vi "CalculateRatio.vi"(0 "ratio":dbl, 1 "Cluster":T1={"increase"=0.01, "min velocity"=0.1, "max velocity"=0.4, "Stop increase"=0.01}, 3 "decrease again":bool=TRUE, 5 "velocity":dbl, 7 "acceleration":dbl, 9 "rep":i32, 11 "downramp":dbl, 12 "stop":bool) -> (4 "ratio out":dbl, 6 "velocity out":dbl, 10 "rep out":i32, 14 "decrease again out":bool)   [LabVIEW 2020]
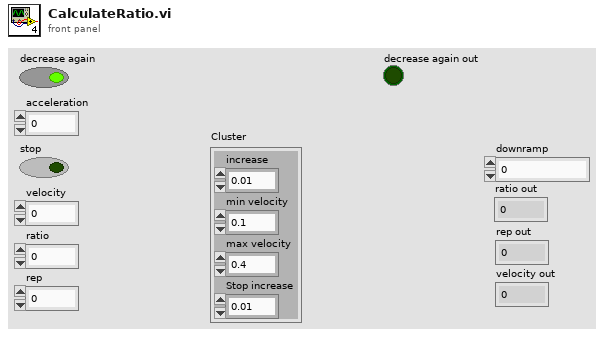
[diagram p1: front panel]
types:
  T1 = cluster{"increase":dbl, "min velocity":dbl, "max velocity":dbl, "Stop increase":dbl}
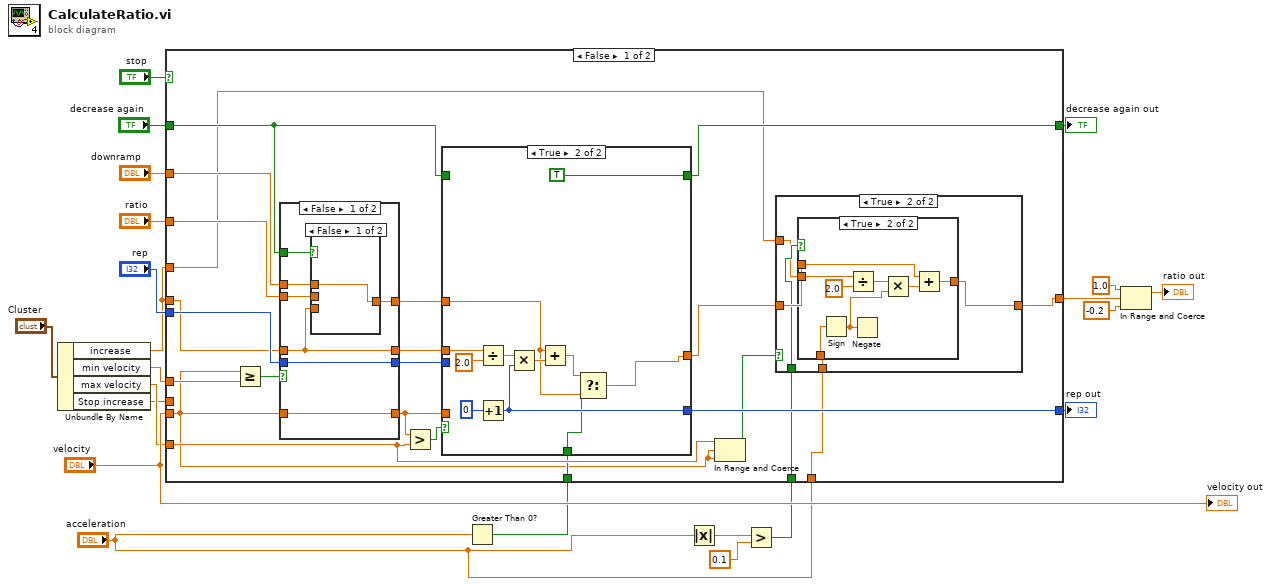
[diagram p0: block diagram]
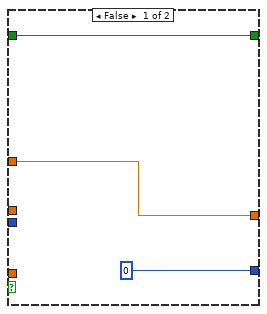
[diagram p4: hidden frame]
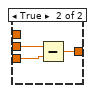
[diagram p5: hidden frame]
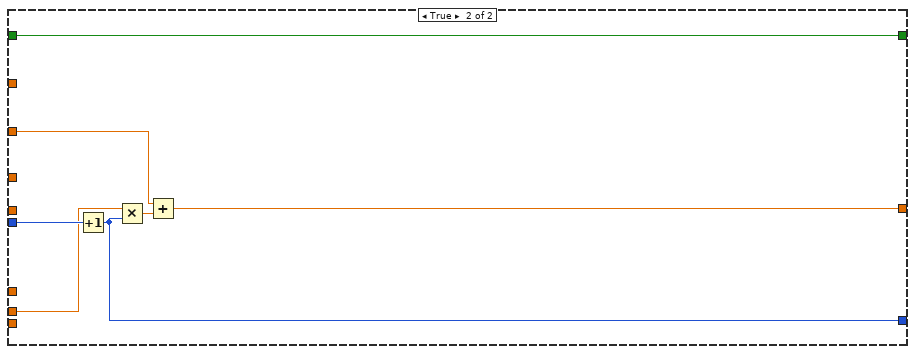
[diagram p7: hidden frame]
diagram:
  n1 = Unbundle By Name("Cluster") -> ("increase"=w1:dbl, "min velocity"=w13:dbl, "max velocity"=w12:dbl, "Stop increase"=w11:dbl)
  n2 = Greater Than 0?(x="acceleration") -> (x > 0?=w6:bool)
  n3 = Absolute Value(x="acceleration") -> (abs(x)=w5:dbl)
  n4 = Greater?(x=w5, y=0.1) -> (0:w3:bool)
  n5 = case shown="False" "stop" {
    tunnel: "velocity" -> [w23 _]
    tunnel: "downramp" -> [w41 _]
    tunnel: "ratio" -> [w40 w96]
    tunnel: [w28 w93] -> w15
    tunnel: "rep" -> [w38 w95]
    tunnel: [w36 w92] -> w9
    tunnel: w1 -> [w35 _]
    tunnel: w13 -> [w34 _]
    tunnel: w12 -> [w31 _]
    tunnel: w11 -> [_ w91]
    tunnel: "decrease again" -> [w32 w90]
    tunnel: [w33 w90] -> w7
    tunnel: w6 -> [w27 _]
    tunnel: w3 -> [w26 _]
    tunnel: "acceleration" -> [w25 _]
    tunnel: w1 -> [w24 _]
    frame False {
      n6 = Greater Or Equal?(x=w23, y=w34) -> (x >= y?=w45:bool)
      n7 = case shown="False" w45 {
        tunnel: w23 -> [w81 w89]
        tunnel: [w81 w89] -> w43
        tunnel: w35 -> [w75 w88]
        tunnel: [w75 w88] -> w42
        tunnel: w41 -> [w79 _]
        tunnel: w40 -> [w76 w87]
        tunnel: [w78 w87] -> w39
        tunnel: w38 -> [w80 w86]
        tunnel: [w80 w86] -> w37
        tunnel: w32 -> [w77 _]
        frame False {
          n8 = case shown="False" w77 {
            tunnel: w79 -> [w82 _]
            tunnel: [w82 w83] -> w78
            tunnel: w76 -> [_ w85]
            tunnel: w75 -> [_ w84]
            frame False {
            }
            frame True {
              n9 = Subtract(x=w85, y=w84) -> (x-y=w83:dbl)
            }
          }
        }
        frame True {
        }
      }
      n10 = Greater?(x=w43, y=w31) -> (0:w44:bool)
      n11 = case shown="True" w44 {
        tunnel: w43 -> [_ _]
        tunnel: w42 -> [_ w74]
        tunnel: [w63 w65] -> w29
        tunnel: w39 -> [w63 w66]
        tunnel: w37 -> [_ _]
        tunnel: [0 w70] -> w36
        tunnel: [w61 TRUE] -> w33
        tunnel: w32 -> [w61 _]
        tunnel: w27 -> [_ w64]
        frame False {
        }
        frame True {
          n12 = Divide(x=w74, y=2.0) -> (x/y=w72:dbl)
          n13 = Increment(x=0) -> (x+1=w70:i32)
          n14 = Multiply(x=w72, y=w70) -> (x*y=w71:dbl)
          n15 = Add(x=w66, y=w71) -> (x+y=w67:dbl)
          n16 = Select(t=w67, s=w64, f=w66) -> (s? t:f=w65:dbl)
        }
      }
      n17 = In Range and Coerce(upper limit=w31, x=w23, lower limit=w23) -> (In Range?=w30:bool)  [unwired: 1 out]
      n18 = case shown="True" w30 {
        tunnel: w29 -> [w46 w51]
        tunnel: [w46 w50] -> w28
        tunnel: w26 -> [_ w49]
        tunnel: w25 -> [_ w48]
        tunnel: w24 -> [_ w47]
        frame False {
        }
        frame True {
          n19 = case shown="True" w49 {
            tunnel: w51 -> [w52 w59]
            tunnel: [w52 w54] -> w50
            tunnel: w48 -> [_ w60]
            tunnel: w47 -> [_ w58]
            frame False {
            }
            frame True {
              n20 = Sign(1:w60) -> (0:w53:dbl)
              n21 = Divide(x=w58, y=2.0) -> (x/y=w56:dbl)
              n22 = Negate(x=w53) -> ()  [unwired: 1 out]
              n23 = Multiply(x=w56, y=w53) -> (x*y=w55:dbl)
              n24 = Add(x=w59, y=w55) -> (x+y=w54:dbl)
            }
          }
        }
      }
    }
    frame True {
      n25 = Increment(x=w95) -> (x+1=w92:i32)
      n26 = Multiply(x=w91, y=w92) -> (x*y=w94:dbl)
      n27 = Add(x=w96, y=w94) -> (x+y=w93:dbl)
    }
  }
  "rep out" <- w9
  "decrease again out" <- w7
  n28 = In Range and Coerce(upper limit=1.0, x=w15, lower limit=-0.2) -> (coerced(x)=→"ratio out":dbl)  [unwired: 1 out]
  "velocity out" <- "velocity"
